vi "Read_Weather_Parameters.vi"(0 "Current PC time":timestamp, 1 "GPS time difference":i32) -> (2 "Current GPS time":timestamp, 3 "Queue overflow?":bool, 4 "Weather data":T1)   [LabVIEW 2013]
uses:
  Globals/DAQ_Mode.vi
  Globals/Weather_Queues.vi
  VantagePro.dll
panel:
  in  "Weather data cluster":T1
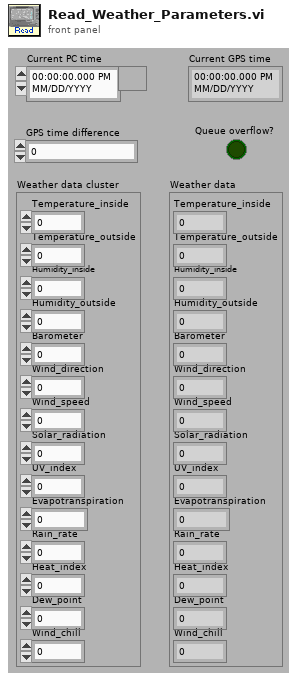
[diagram p1: front panel]
types:
  T1 = cluster{"Temperature_inside":sgl, "Temperature_outside":sgl, "Humidity_inside":sgl, "Humidity_outside":sgl, "Barometer":sgl, "Wind_direction":sgl, "Wind_speed":sgl, "Solar_radiation":sgl, "UV_index":sgl, "Evapotranspiration":sgl, "Rain_rate":sgl, "Heat_index":sgl, "Dew_point":sgl, "Wind_chill":sgl}
  T2 = cluster{"Weather data (5s)":refnum<queue>, "Database queue":refnum<queue>, "Message queue":refnum<queue>, "Settings queue":refnum<queue>, "60 mins data queue":refnum<queue>, "48 hrs data queue":refnum<queue>}
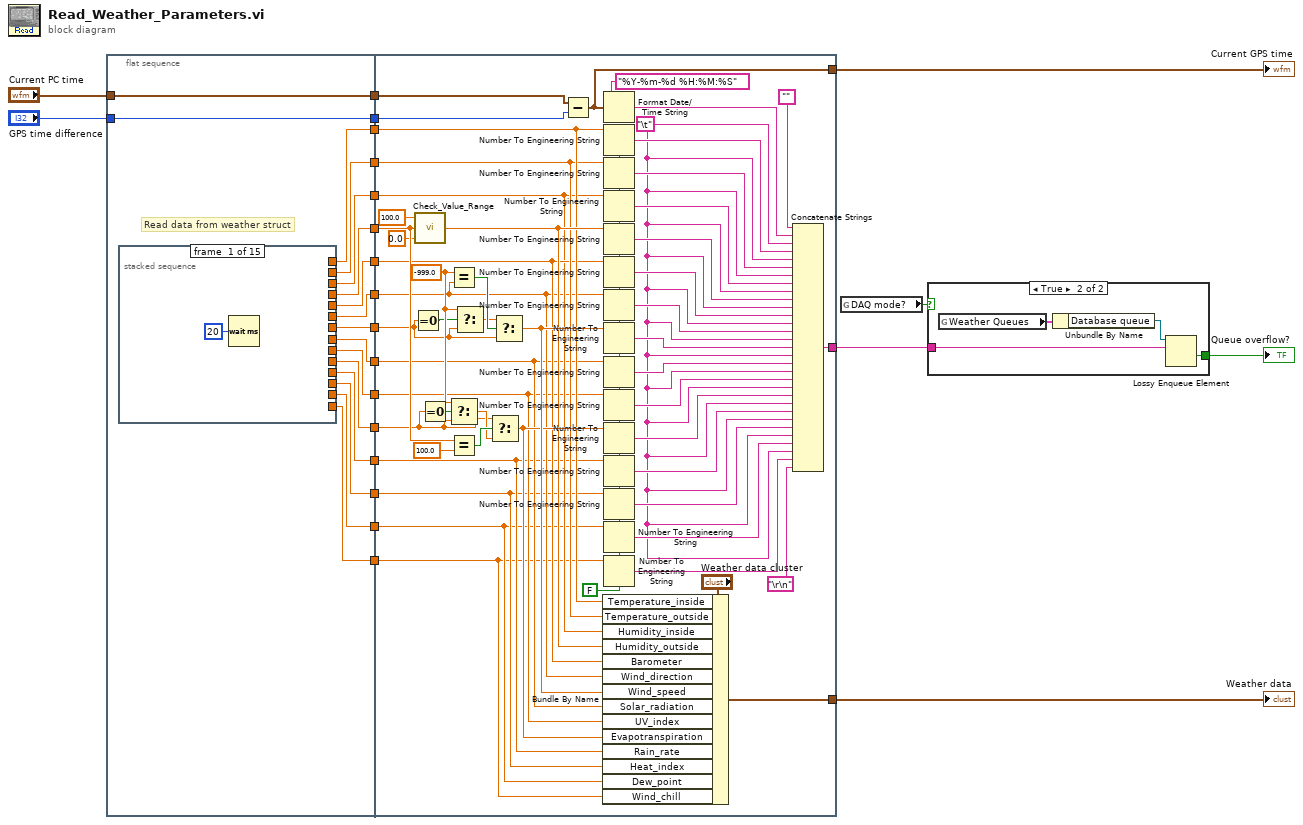
[diagram p0: block diagram]
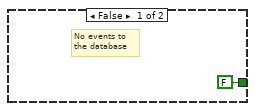
[diagram p2: hidden frame]
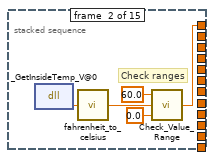
[diagram p3: hidden frame]
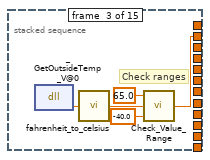
[diagram p4: hidden frame]
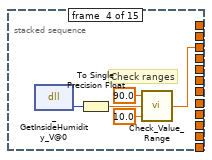
[diagram p5: hidden frame]
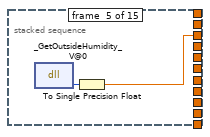
[diagram p6: hidden frame]
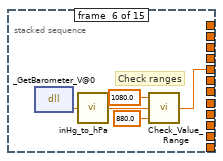
[diagram p7: hidden frame]
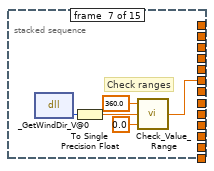
[diagram p8: hidden frame]
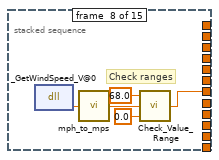
[diagram p9: hidden frame]
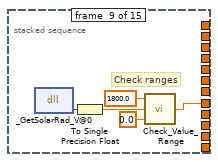
[diagram p10: hidden frame]
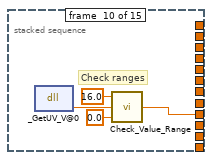
[diagram p11: hidden frame]
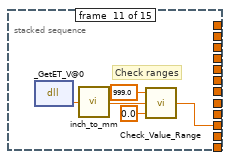
[diagram p12: hidden frame]
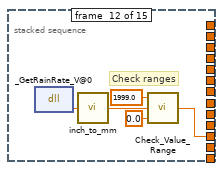
[diagram p13: hidden frame]
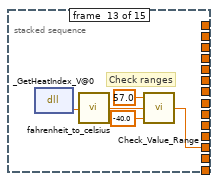
[diagram p14: hidden frame]
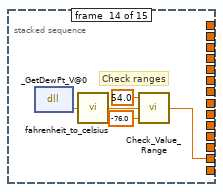
[diagram p15: hidden frame]
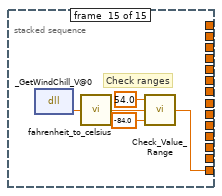
[diagram p16: hidden frame]
diagram:
  n1 = flat-sequence {
    tunnel: [w28] -> w16
    tunnel: [w31] -> w15
    tunnel: [w30] -> w14
    tunnel: [w39] -> w13
    tunnel: [w38] -> w12
    tunnel: [w29] -> w11
    tunnel: [w27] -> w10
    tunnel: [w25] -> w9
    tunnel: [w24] -> w8
    tunnel: "Current PC time" -> [w39]
    tunnel: "GPS time difference" -> [w38]
    tunnel: [w37] -> w7
    tunnel: [w36] -> w6
    tunnel: [w35] -> w5
    tunnel: [w34] -> w4
    tunnel: [w33] -> w3
    tunnel: [w32] -> w2
    tunnel: [w26] -> w1
    tunnel: w16 -> [w120]
    tunnel: w15 -> [w123]
    tunnel: w14 -> [w122]
    tunnel: w13 -> [w111]
    tunnel: w12 -> [w112]
    tunnel: w11 -> [w121]
    tunnel: w10 -> [w119]
    tunnel: w9 -> [w117]
    tunnel: w8 -> [w116]
    tunnel: w7 -> [w128]
    tunnel: w6 -> [w127]
    tunnel: w5 -> [w125]
    tunnel: w4 -> [w134]
    tunnel: w3 -> [w126]
    tunnel: w2 -> [w124]
    tunnel: w1 -> [w118]
    tunnel: [w159] -> w19
    tunnel: [w158] -> w23
    tunnel: [w109] -> w20
    frame #0 {
      # "Read data from weather struct"
      n2 = stacked-sequence {
        tunnel: [_ w41 _ _ _ _ _ _ _ _ _ _ _ _ _] -> w37
        tunnel: [_ _ w46 _ _ _ _ _ _ _ _ _ _ _ _] -> w36
        tunnel: [_ _ _ w51 _ _ _ _ _ _ _ _ _ _ _] -> w35
        tunnel: [_ _ _ _ w56 _ _ _ _ _ _ _ _ _ _] -> w34
        tunnel: [_ _ _ _ _ w60 _ _ _ _ _ _ _ _ _] -> w33
        tunnel: [_ _ _ _ _ _ w63 _ _ _ _ _ _ _ _] -> w32
        tunnel: [_ _ _ _ _ _ _ w68 _ _ _ _ _ _ _] -> w31
        tunnel: [_ _ _ _ _ _ _ _ w74 _ _ _ _ _ _] -> w30
        tunnel: [_ _ _ _ _ _ _ _ _ w78 _ _ _ _ _] -> w29
        tunnel: [_ _ _ _ _ _ _ _ _ _ w82 _ _ _ _] -> w28
        tunnel: [_ _ _ _ _ _ _ _ _ _ _ w87 _ _ _] -> w27
        tunnel: [_ _ _ _ _ _ _ _ _ _ _ _ w92 _ _] -> w26
        tunnel: [_ _ _ _ _ _ _ _ _ _ _ _ _ w97 _] -> w25
        tunnel: [_ _ _ _ _ _ _ _ _ _ _ _ _ _ w102] -> w24
        frame #0 {
          n3 = Wait (ms)(milliseconds to wait=u32 20 ("millisecond multiple")) -> ()  [unwired: 1 out]
        }
        frame #1 {
          # "Check ranges"
          n4 = dll-call lib="C:/Users/Bob van Eijk/Desktop/LabView Projects 13/HiSPARC Weather Station/Develop/VantagePro.dll" fn="_GetInsideTemp_V@0" label="Get InsideTemperature"() -> ("return type"=w42:sgl)  [unwired: 3 in, 2 out]
          n5 = call "fahrenheit_to_celsius.vi"("Fahrenheit"=w42) -> ("Celsius"=w45:sgl)
          n6 = call "Check_Value_Range.vi"("Min"=sgl 0.0, "Data in"=w45, "Max"=sgl 60.0) -> ("Data out"=w41:sgl)
        }
        frame #2 {
          # "Check ranges"
          n7 = dll-call lib="C:/Users/Bob van Eijk/Desktop/LabView Projects 13/HiSPARC Weather Station/Develop/VantagePro.dll" fn="_GetOutsideTemp_V@0" label="Get Outside Temperature"() -> ("return type"=w47:sgl)  [unwired: 3 in, 2 out]
          n8 = call "fahrenheit_to_celsius.vi"("Fahrenheit"=w47) -> ("Celsius"=w50:sgl)
          n9 = call "Check_Value_Range.vi"("Min"=sgl -40.0, "Data in"=w50, "Max"=sgl 65.0) -> ("Data out"=w46:sgl)
        }
        frame #3 {
          # "Check ranges"
          n10 = dll-call lib="C:/Users/Bob van Eijk/Desktop/LabView Projects 13/HiSPARC Weather Station/Develop/VantagePro.dll" fn="_GetInsideHumidity_V@0" label="Get Inside Humidity"() -> ("return type"=w53:i16)  [unwired: 3 in, 2 out]
          n11 = To Single Precision Float(number=w53) -> (single precision float=w52:sgl)
          n12 = call "Check_Value_Range.vi"("Min"=sgl 10.0, "Data in"=w52, "Max"=sgl 90.0) -> ("Data out"=w51:sgl)
        }
        frame #4 {
          n13 = dll-call lib="C:/Users/Bob van Eijk/Desktop/LabView Projects 13/HiSPARC Weather Station/Develop/VantagePro.dll" fn="_GetOutsideHumidity_V@0" label="Get Outside Humidity"() -> ("return type"=w57:i16)  [unwired: 3 in, 2 out]
          n14 = To Single Precision Float(number=w57) -> (single precision float=w56:sgl)
        }
        frame #5 {
          # "Check ranges"
          n15 = dll-call lib="C:/Users/Bob van Eijk/Desktop/LabView Projects 13/HiSPARC Weather Station/Develop/VantagePro.dll" fn="_GetBarometer_V@0" label="Get Barometer"() -> ("return type"=w59:sgl)  [unwired: 3 in, 2 out]
          n16 = call "inHg_to_hPa.vi"("inHg"=w59) -> ("hPa"=w58:sgl)
          n17 = call "Check_Value_Range.vi"("Min"=sgl 880.0, "Data in"=w58, "Max"=sgl 1080.0) -> ("Data out"=w60:sgl)
        }
        frame #6 {
          # "Check ranges"
          n18 = dll-call lib="C:/Users/Bob van Eijk/Desktop/LabView Projects 13/HiSPARC Weather Station/Develop/VantagePro.dll" fn="_GetWindDir_V@0" label="Get Wind Direction"() -> ("return type"=w65:i16)  [unwired: 3 in, 2 out]
          n19 = To Single Precision Float(number=w65) -> (single precision float=w64:sgl)
          n20 = call "Check_Value_Range.vi"("Min"=sgl 0.0, "Data in"=w64, "Max"=sgl 360.0) -> ("Data out"=w63:sgl)
        }
        frame #7 {
          # "Check ranges"
          n21 = dll-call lib="C:/Users/Bob van Eijk/Desktop/LabView Projects 13/HiSPARC Weather Station/Develop/VantagePro.dll" fn="_GetWindSpeed_V@0" label="Get Wind Speed"() -> ("return type"=w69:sgl)  [unwired: 3 in, 2 out]
          n22 = call "mph_to_mps.vi"("Miles/hour"=w69) -> ("Meter/second"=w70:sgl)
          n23 = call "Check_Value_Range.vi"("Min"=sgl 0.0, "Data in"=w70, "Max"=sgl 68.0) -> ("Data out"=w68:sgl)
        }
        frame #8 {
          # "Check ranges"
          n24 = dll-call lib="C:/Users/Bob van Eijk/Desktop/LabView Projects 13/HiSPARC Weather Station/Develop/VantagePro.dll" fn="_GetSolarRad_V@0" label="Get Solar Radiation"() -> ("return type"=w73:i16)  [unwired: 3 in, 2 out]
          n25 = To Single Precision Float(number=w73) -> (single precision float=w75:sgl)
          n26 = call "Check_Value_Range.vi"("Min"=sgl 0.0, "Data in"=w75, "Max"=sgl 1800.0) -> ("Data out"=w74:sgl)
        }
        frame #9 {
          # "Check ranges"
          n27 = dll-call lib="C:/Users/Bob van Eijk/Desktop/LabView Projects 13/HiSPARC Weather Station/Develop/VantagePro.dll" fn="_GetUV_V@0" label="Get UV"() -> ("return type"=w79:sgl)  [unwired: 3 in, 2 out]
          n28 = call "Check_Value_Range.vi"("Min"=sgl 0.0, "Data in"=w79, "Max"=sgl 16.0) -> ("Data out"=w78:sgl)
        }
        frame #10 {
          # "Check ranges"
          n29 = dll-call lib="C:/Users/Bob van Eijk/Desktop/LabView Projects 13/HiSPARC Weather Station/Develop/VantagePro.dll" fn="_GetET_V@0" label="Get ET"() -> ("return type"=w83:sgl)  [unwired: 3 in, 2 out]
          n30 = call "inch_to_mm.vi"("inches"=w83) -> ("mm"=w84:sgl)
          n31 = call "Check_Value_Range.vi"("Min"=sgl 0.0, "Data in"=w84, "Max"=sgl 999.0) -> ("Data out"=w82:sgl)
        }
        frame #11 {
          # "Check ranges"
          n32 = dll-call lib="C:/Users/Bob van Eijk/Desktop/LabView Projects 13/HiSPARC Weather Station/Develop/VantagePro.dll" fn="_GetRainRate_V@0" label="Get Rain Rate"() -> ("return type"=w90:sgl)  [unwired: 3 in, 2 out]
          n33 = call "inch_to_mm.vi"("inches"=w90) -> ("mm"=w91:sgl)
          n34 = call "Check_Value_Range.vi"("Min"=sgl 0.0, "Data in"=w91, "Max"=sgl 1999.0) -> ("Data out"=w87:sgl)
        }
        frame #12 {
          # "Check ranges"
          n35 = dll-call lib="C:/Users/Bob van Eijk/Desktop/LabView Projects 13/HiSPARC Weather Station/Develop/VantagePro.dll" fn="_GetHeatIndex_V@0" label="Get Heat Index"() -> ("return type"=w95:sgl)  [unwired: 3 in, 2 out]
          n36 = call "fahrenheit_to_celsius.vi"("Fahrenheit"=w95) -> ("Celsius"=w96:sgl)
          n37 = call "Check_Value_Range.vi"("Min"=sgl -40.0, "Data in"=w96, "Max"=sgl 57.0) -> ("Data out"=w92:sgl)
        }
        frame #13 {
          # "Check ranges"
          n38 = dll-call lib="C:/Users/Bob van Eijk/Desktop/LabView Projects 13/HiSPARC Weather Station/Develop/VantagePro.dll" fn="_GetDewPt_V@0" label="Get Dew Point"() -> ("return type"=w99:sgl)  [unwired: 3 in, 2 out]
          n39 = call "fahrenheit_to_celsius.vi"("Fahrenheit"=w99) -> ("Celsius"=w98:sgl)
          n40 = call "Check_Value_Range.vi"("Min"=sgl -76.0, "Data in"=w98, "Max"=sgl 54.0) -> ("Data out"=w97:sgl)
        }
        frame #14 {
          # "Check ranges"
          n41 = dll-call lib="C:/Users/Bob van Eijk/Desktop/LabView Projects 13/HiSPARC Weather Station/Develop/VantagePro.dll" fn="_GetWindChill_V@0" label="Get Wind Chill"() -> ("return type"=w105:sgl)  [unwired: 3 in, 2 out]
          n42 = call "fahrenheit_to_celsius.vi"("Fahrenheit"=w105) -> ("Celsius"=w106:sgl)
          n43 = call "Check_Value_Range.vi"("Min"=sgl -84.0, "Data in"=w106, "Max"=sgl 54.0) -> ("Data out"=w102:sgl)
        }
      }
    }
    frame #1 {
      w107 = FALSE
      w132 = sgl -999.0 ("y")
      w113 = "\t"
      n44 = Equal To 0?(x=w123) -> (x = 0?=w130:bool)
      n45 = call "Check_Value_Range.vi"("Min"=sgl 0.0, "Data in"=w134, "Max"=sgl 100.0) -> ("Data out"=w133:sgl)
      n46 = Equal To 0?(x=w120) -> (x = 0?=w138:bool)
      n47 = Equal?(x=w132, y=w124) -> (x = y?=w140:bool)
      n48 = Select(t=w132, s=w138, f=w120) -> (s? t:f=w135:sgl)
      n49 = Equal?(x=w134, y=sgl 100.0) -> (x = y?=w139:bool)
      n50 = Select(t=w132, s=w130, f=w123) -> (s? t:f=w131:sgl)
      n51 = Select(t=w120, s=w139, f=w135) -> (s? t:f=w137:sgl)
      n52 = Select(t=w131, s=w140, f=w123) -> (s? t:f=w141:sgl)
      n53 = Subtract(x=w111, y=w112) -> (x-y=w109:timestamp)
      n54 = Bundle By Name(cluster="Weather data cluster", "Temperature_inside"=w128, "Temperature_outside"=w127, "Humidity_inside"=w125, "Humidity_outside"=w133, "Barometer"=w126, "Wind_direction"=w124, "Wind_speed"=w141, "Solar_radiation"=w122, "UV_index"=w121, "Evapotranspiration"=w137, "Rain_rate"=w119, "Heat_index"=w118, "Dew_point"=w117, "Wind_chill"=w116) -> (w158:T1)
      n55 = Format Date/Time String(time format string (%c)="%Y-%m-%d %H:%M:%S", seconds (now)=w109) -> (date/time string=w108:string)  [unwired: 1 out]
      n56 = Number To Engineering String(1:w107, 4:w128) -> (0:w145:string)  [unwired: 2 out]
      n57 = Number To Engineering String(1:w107, 4:w127) -> (0:w144:string)  [unwired: 2 out]
      n58 = Number To Engineering String(1:w107, 4:w125) -> (0:w150:string)  [unwired: 2 out]
      n59 = Number To Engineering String(1:w107, 4:w133) -> (0:w151:string)  [unwired: 2 out]
      n60 = Number To Engineering String(1:w107, 4:w126) -> (0:w152:string)  [unwired: 2 out]
      n61 = Number To Engineering String(1:w107, 4:w124) -> (0:w147:string)  [unwired: 2 out]
      n62 = Number To Engineering String(1:w107, 4:w141) -> (0:w146:string)  [unwired: 2 out]
      n63 = Number To Engineering String(1:w107, 4:w122) -> (0:w153:string)  [unwired: 2 out]
      n64 = Number To Engineering String(1:w107, 4:w121) -> (0:w143:string)  [unwired: 2 out]
      n65 = Number To Engineering String(1:w107, 4:w137) -> (0:w142:string)  [unwired: 2 out]
      n66 = Number To Engineering String(1:w107, 4:w119) -> (0:w154:string)  [unwired: 2 out]
      n67 = Number To Engineering String(1:w107, 4:w118) -> (0:w155:string)  [unwired: 2 out]
      n68 = Number To Engineering String(1:w107, 4:w117) -> (0:w156:string)  [unwired: 2 out]
      n69 = Number To Engineering String(1:w107, 4:w116) -> (0:w157:string)  [unwired: 2 out]
      n70 = Concatenate Strings("", w108, w113, w145, w113, w144, w113, w150, w113, w151, w113, w152, w113, w147, w113, w146, w113, w153, w113, w143, w113, w142, w113, w154, w113, w155, w113, w156, w113, w157, "\r\n") -> (w159:string)
    }
  }
  n71 = global read "DAQ_Mode.vi" "DAQ mode?"() -> (w18:bool)
  n72 = case shown="True" w18 {
    tunnel: w19 -> [_ w164]
    tunnel: [FALSE ("overflow?") w163] -> w17
    frame False {
      # "No events to\nthe database"
    }
    frame True {
      n73 = global read "Weather_Queues.vi" "Weather Queues"() -> (w162:T2)
      n74 = Unbundle By Name(w162) -> ("Database queue"=w161:refnum<queue>)
      n75 = Lossy Enqueue Element(queue=w161, element=w164) -> (overflow?=w163:bool)  [unwired: 1 in, 3 out]
    }
  }
  "Queue overflow?" <- w17
  "Current GPS time" <- w20
  "Weather data" <- w23
